vi "PH_PSDBWriter.update Information.vi"(1 "Instance ID":i32, 2 "Shot #":i32, 3 "Subsystem":T2 caption="PHELIX Subsysteme" items=["Miscellaneous", "fs-Frontend", "ns-Frontend", "PreAmp", "MainAmp", "MAS", "COS", "Beamline", "Experiment Laserbay", "Experiment Laserlabor", "Experiment Z6", "Timing", "Pulsed Power"], 4 "Data Status":T1 items=["no info", "no Data collection", "no problem", "Error getting the ID", "Error writing Data", "Error getting the subsystem", "Error getting the Shot ID", "Error getting the Shot Types", "Error getting the Experiments", "Error verifying wanted Shottype", "Error verifying wanted Experiment"], 5 "error in":errorcluster, 6 "GUI Ref PSDB Status":refnum<vi>, 7 "BSDB Status Service ID":i32, 9 "PSDB Error Code":i32) -> (19 "error out":errorcluster)   [LabVIEW 2014, in "PH_PSDBWriter.lvlib"]
doc: "This VI updates the data service and sets the related GUI element."
uses:
  PH_PSDBWriter.lvlib
  PH_PSDBWriter.PHELIX-Subsystems.ctl
  PH_PSDBWriter.Data Status.ctl
  PH_Common/PH_Common.lvlib
panel:
  in  "Data Status Dummy":T1 items=["no info", "no Data collection", "no problem", "Error getting the ID", "Error writing Data", "Error getting the subsystem", "Error getting the Shot ID", "Error getting the Shot Types", "Error getting the Experiments", "Error verifying wanted Shottype", "Error verifying wanted Experiment"]
  in  "Subsystem Dummy":T2 caption="PHELIX Subsysteme" items=["Miscellaneous", "fs-Frontend", "ns-Frontend", "PreAmp", "MainAmp", "MAS", "COS", "Beamline", "Experiment Laserbay", "Experiment Laserlabor", "Experiment Z6", "Timing", "Pulsed Power"]
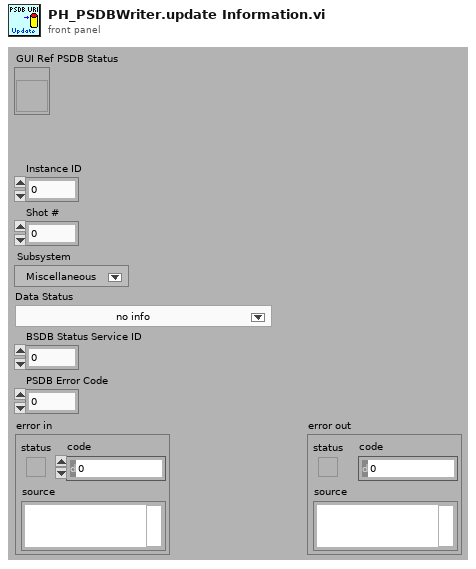
[diagram p1: front panel]
types:
  T1 = typedef "PH_PSDBWriter.lvlib/PH_PSDBWriter.Data Status.ctl" = i16
  T2 = typedef "PH_PSDBWriter.lvlib/PH_PSDBWriter.PHELIX-Subsystems.ctl" = i32
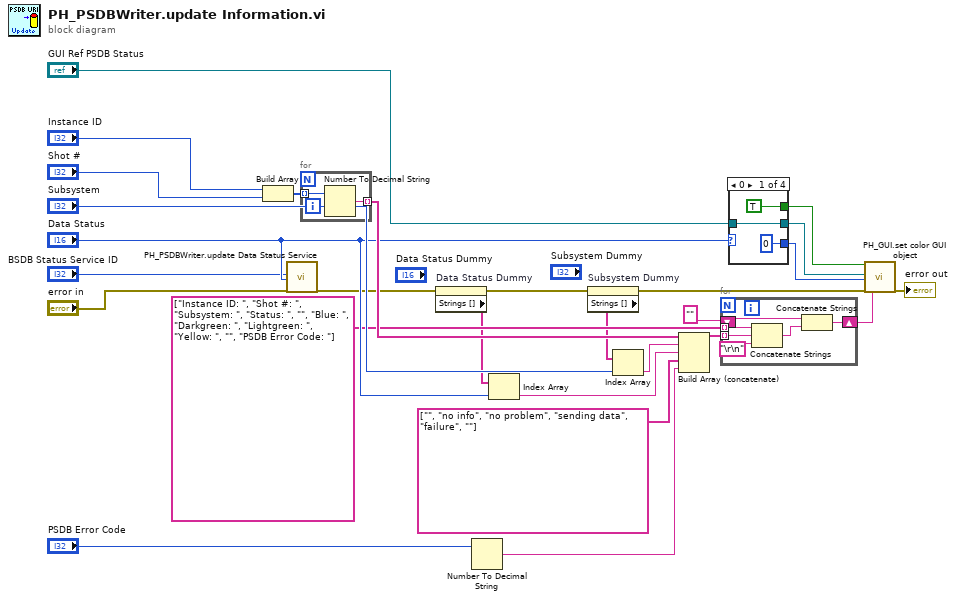
[diagram p0: block diagram]
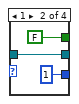
[diagram p2: hidden frame]
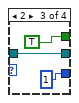
[diagram p3: hidden frame]
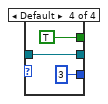
[diagram p4: hidden frame]
diagram:
  n1 = Build Array("Instance ID", "Shot #") -> (w11:i32[])
  n2 = call "PH_PSDBWriter.update Data Status Service.vi"("Service ID"="BSDB Status Service ID", "Data Status"="Data Status", "error in (no error)"="error in") -> ("error out"=w3:errorcluster)  [unwired: 16 in]
  n3 = for {
    tunnel: w11 -> [w29] mode=indexing
    tunnel: [w28] -> w27 mode=indexing
    n4 = Number To Decimal String(number=w29) -> (decimal integer string=w28:string)  [unwired: 1 in]
  }
  n5 = property on="Data Status Dummy" class="Ring (strict)"(error in=w3) -> (error out=w2:errorcluster, "Strings []"=w5:string[])  [unwired: 1 in, 1 out]
  n6 = Number To Decimal String(number="PSDB Error Code") -> (decimal integer string=w24:string)  [unwired: 1 in]
  n7 = Index Array(array=w5, index="Data Status") -> (element=w9:string)
  n8 = property on="Subsystem Dummy" class="Ring (strict)"(error in=w2) -> (error out=w1:errorcluster, "Strings []"=w4:string[])  [unwired: 1 in, 1 out]
  n9 = Index Array(array=w4, index="Subsystem") -> (element=w10:string)
  n10 = Build Array (concatenate)(w27, w10, w9, string[] ["", "no info", "no problem", "sending data", "failure", ""], w24) -> (w8:string[])
  n11 = for {
    tunnel: string[] ["Instance ID: ", "Shot #: ", "Subsystem: ", "Status: ", "", "Blue: ", "Darkgreen: ", "Lightgreen: ", "Yellow: ", "", "PSDB Error Code: "] -> [w31] mode=indexing
    shift-right: [w34] -> w26
    shift-left: "" -> [w35]
    tunnel: w8 -> [w32] mode=indexing
    n12 = Concatenate Strings(w31, w32, "\r\n") -> (w30:string)
    n13 = Concatenate Strings(w35, w30) -> (w34:string)
  }
  n14 = case shown="0" "Data Status" {
    tunnel: [TRUE FALSE TRUE TRUE] -> w16
    tunnel: [w37 w40 w43 w46] -> w14
    tunnel: "GUI Ref PSDB Status" -> [w37 w40 w43 w46]
    tunnel: [0 ("State") 1 ("State") 1 ("State") 3 ("State")] -> w15
    frame 0 {
    }
    frame 1 {
    }
    frame 2 {
    }
    frame Default {
    }
  }
  n15 = call "PH_GUI.set color GUI object.vi"("Visible? (true)"=w16, "GUI object Ref"=w14, "State"=w15, "error in (no error)"=w1, "Tip Strip (N/A)"=w26) -> ("error out"=→"error out":errorcluster)  [unwired: 14 in]
